vi "Terminals - Filter invalid Terms.vi"(11 "Terms[]":refnum<vi>[](array[refnum])) -> (3 "Terms[] out":refnum<vi>[](array[refnum]))   [LabVIEW 2017, in "csmHelper-Terminals.lvlib"]
uses:
  csmHelper-Terminals.lvlib
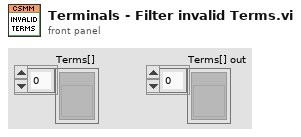
[diagram p1: front panel]
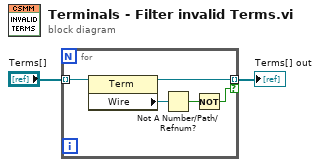
[diagram p0: block diagram]
diagram:
  n1 = for {
    tunnel: "Terms[]" -> [w7] mode=indexing
    tunnel: [w5] -> w1 mode=indexing if=w4
    n2 = property class="Term"(reference=w7) -> (reference out=w5:refnum<vi>, "Wire"=w6:refnum<vi>)  [unwired: 1 in, 1 out]
    n3 = Not A Number/Path/Refnum?(number/path/refnum=w6) -> (NaN/Path/Refnum?=w3:bool)
    n4 = Not(x=w3) -> (.not. x?=w4:bool)
  }
  "Terms[] out" <- w1
